vi "Open Connection to All - String Type Array.vi"(8 "Error In":errorcluster, 10 "Type array":string[](array[string]), 11 "URL array":string[](array[string])) -> (0 "Error Out":errorcluster, 2 "Error Status":bool, 3 "Array of SV Refnums":refnum<k21>[](array[refnum]))   [LabVIEW 2014]
doc: "<B>Copyright</B>: (c) 2015 MHWirth. All rights reserved.\n\nThis VI opens connection to all shared variables that are specified using URL and Type arrays.\n\nIf the type is unknown (Error 7001) or read variable function is errorenous, the loop stops and Error Status is True."
panel:
  out "Status":string
  out "Number of Deployed SV":i32
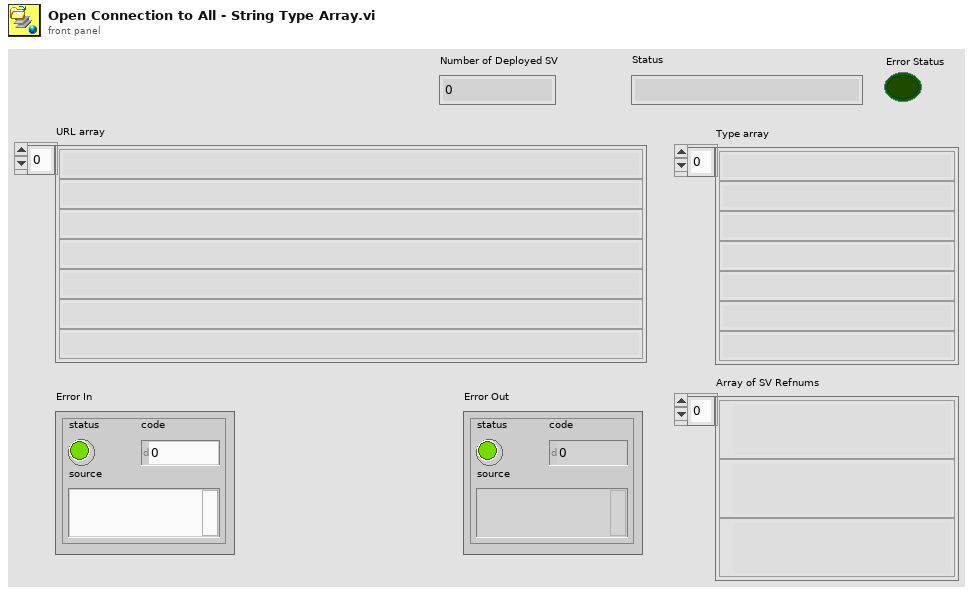
[diagram p1: front panel]
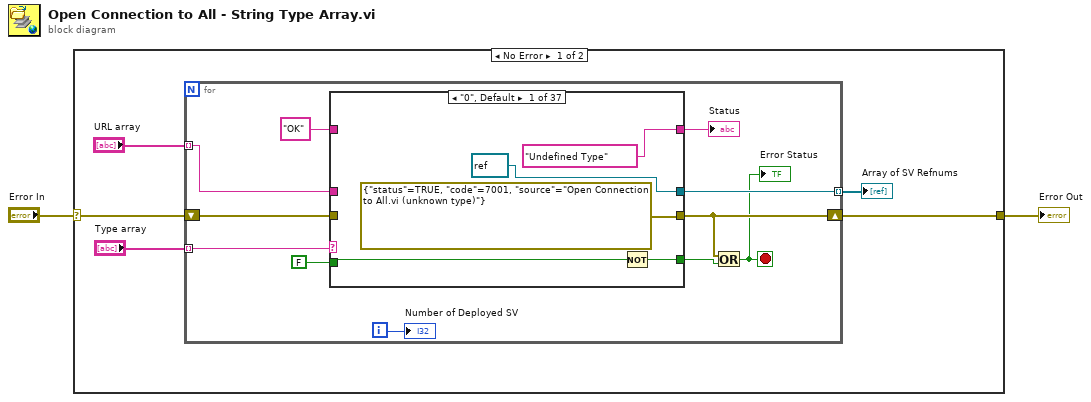
[diagram p0: block diagram]
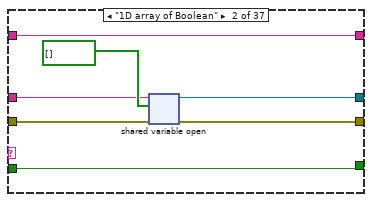
[diagram p2: hidden frame]
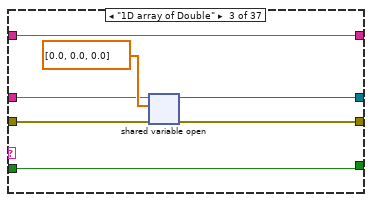
[diagram p3: hidden frame]
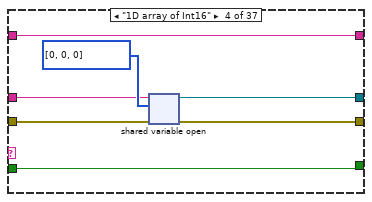
[diagram p4: hidden frame]
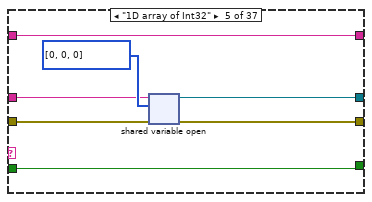
[diagram p5: hidden frame]
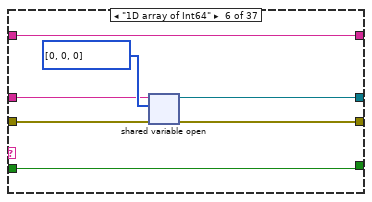
[diagram p6: hidden frame]
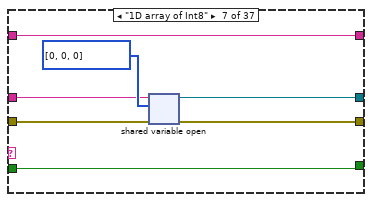
[diagram p7: hidden frame]
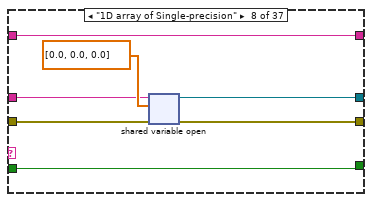
[diagram p8: hidden frame]
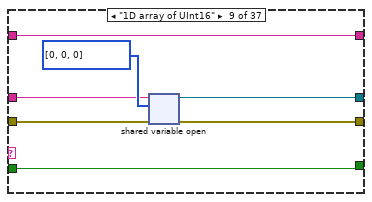
[diagram p9: hidden frame]
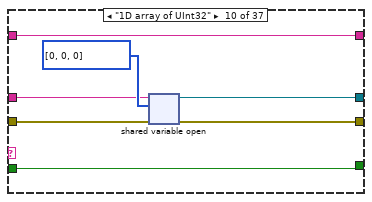
[diagram p10: hidden frame]
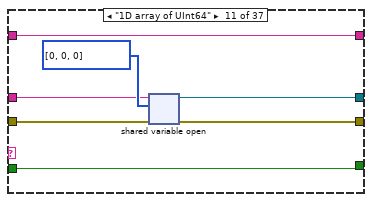
[diagram p11: hidden frame]
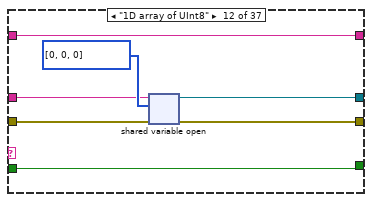
[diagram p12: hidden frame]
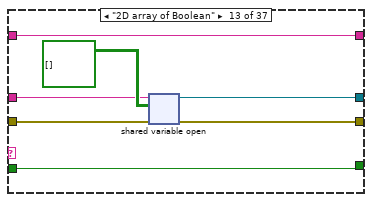
[diagram p13: hidden frame]
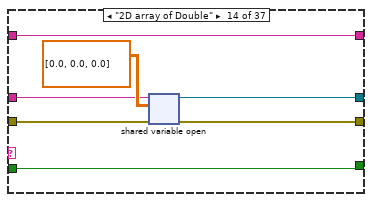
[diagram p14: hidden frame]
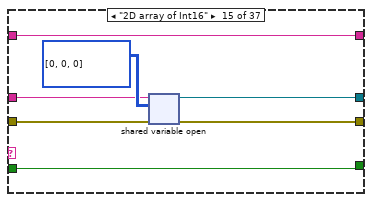
[diagram p15: hidden frame]
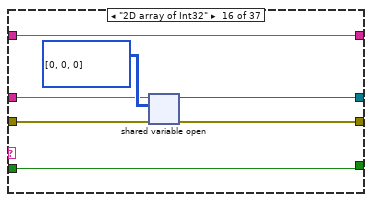
[diagram p16: hidden frame]
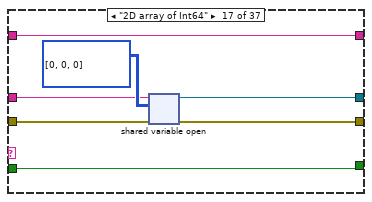
[diagram p17: hidden frame]
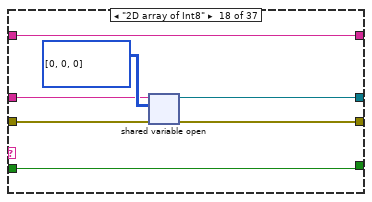
[diagram p18: hidden frame]
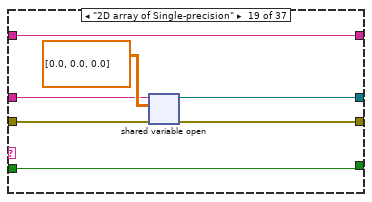
[diagram p19: hidden frame]
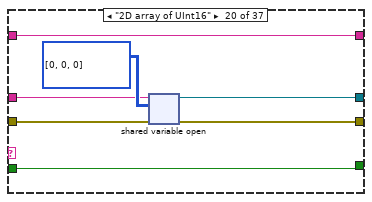
[diagram p20: hidden frame]
diagram:
  n1 = case shown="No Error" "Error In" {
    selector: "Error In" -> [w7 w276]
    tunnel: [w6 w276] -> w1
    frame No Error {
      n2 = for {
        shift-right: [w9] -> w6
        shift-left: w7 -> [w18]
        tunnel: "Type array" -> [w13] mode=indexing
        tunnel: "URL array" -> [w12] mode=indexing
        tunnel: [w11] -> w3 mode=indexing
        i -> [w17]
        stop <- w8 stop-if-true
        n3 = case shown="\"0\", Default" w13 {
          tunnel: w18 -> [_ w29 w36 w43 w50 w57 w64 w71 w78 w85 w92 w99 w106 w113 w120 w127 w134 w141 w148 w155 w162 w169 w176 w183 w191 w197 w204 w211 w218 w225 w232 w239 w246 w253 w260 w267 w274]
          tunnel: [errorcluster {"status"=TRUE, "code"=7001, "source"="Open Connection to All.vi (unknown type)"} ("error constant") w26 w32 w40 w47 w54 w61 w68 w75 w82 w89 w96 w103 w110 w117 w124 w131 w138 w145 w152 w159 w166 w173 w180 w187 w194 w201 w208 w215 w222 w229 w236 w243 w250 w257 w264 w271] -> w9
          tunnel: ["Undefined Type" w28 w35 w42 w49 w56 w63 w70 w77 w84 w91 w98 w105 w112 w119 w126 w133 w140 w147 w154 w161 w168 w175 w182 w190 w196 w203 w210 w217 w224 w231 w238 w245 w252 w259 w266 w273] -> w16
          tunnel: "OK" -> [_ w28 w35 w42 w49 w56 w63 w70 w77 w84 w91 w98 w105 w112 w119 w126 w133 w140 w147 w154 w161 w168 w175 w182 w190 w196 w203 w210 w217 w224 w231 w238 w245 w252 w259 w266 w273]
          tunnel: FALSE -> [w22 w27 w34 w41 w48 w55 w62 w69 w76 w83 w90 w97 w104 w111 w118 w125 w132 w139 w146 w153 w160 w167 w174 w181 w189 w195 w202 w209 w216 w223 w230 w237 w244 w251 w258 w265 w272]
          tunnel: [w21 w27 w34 w41 w48 w55 w62 w69 w76 w83 w90 w97 w104 w111 w118 w125 w132 w139 w146 w153 w160 w167 w174 w181 w189 w195 w202 w209 w216 w223 w230 w237 w244 w251 w258 w265 w272] -> w10
          tunnel: w12 -> [_ w25 w33 w39 w46 w53 w60 w67 w74 w81 w88 w95 w102 w109 w116 w123 w130 w137 w144 w151 w158 w165 w172 w179 w186 w193 w200 w207 w214 w221 w228 w235 w242 w249 w256 w263 w270]
          tunnel: [refnum<k21> refnum w24 w31 w38 w45 w52 w59 w66 w73 w80 w87 w94 w101 w108 w115 w122 w129 w136 w143 w150 w157 w164 w171 w178 w185 w192 w199 w206 w213 w220 w227 w234 w241 w248 w255 w262 w269] -> w11
          frame "0", Default {
            n4 = Not(x=w22) -> (.not. x?=w21:bool)
          }
          frame "1D array of Boolean" {
            n5 = shared-variable-open(w25, w29, bool[] []) -> (w24:refnum<k21>, w26:errorcluster)  [unwired: 1 in]
          }
          frame "1D array of Double" {
            n6 = shared-variable-open(w33, w36, dbl[] [0.0, 0.0, 0.0]) -> (w31:refnum<k21>, w32:errorcluster)  [unwired: 1 in]
          }
          frame "1D array of Int16" {
            n7 = shared-variable-open(w39, w43, i16[] [0, 0, 0]) -> (w38:refnum<k21>, w40:errorcluster)  [unwired: 1 in]
          }
          frame "1D array of Int32" {
            n8 = shared-variable-open(w46, w50, i32[] [0, 0, 0]) -> (w45:refnum<k21>, w47:errorcluster)  [unwired: 1 in]
          }
          frame "1D array of Int64" {
            n9 = shared-variable-open(w53, w57, i64[] [0, 0, 0]) -> (w52:refnum<k21>, w54:errorcluster)  [unwired: 1 in]
          }
          frame "1D array of Int8" {
            n10 = shared-variable-open(w60, w64, i8[] [0, 0, 0]) -> (w59:refnum<k21>, w61:errorcluster)  [unwired: 1 in]
          }
          frame "1D array of Single-precision" {
            n11 = shared-variable-open(w67, w71, sgl[] [0.0, 0.0, 0.0]) -> (w66:refnum<k21>, w68:errorcluster)  [unwired: 1 in]
          }
          frame "1D array of UInt16" {
            n12 = shared-variable-open(w74, w78, u16[] [0, 0, 0]) -> (w73:refnum<k21>, w75:errorcluster)  [unwired: 1 in]
          }
          frame "1D array of UInt32" {
            n13 = shared-variable-open(w81, w85, u32[] [0, 0, 0]) -> (w80:refnum<k21>, w82:errorcluster)  [unwired: 1 in]
          }
          frame "1D array of UInt64" {
            n14 = shared-variable-open(w88, w92, u64[] [0, 0, 0]) -> (w87:refnum<k21>, w89:errorcluster)  [unwired: 1 in]
          }
          frame "1D array of UInt8" {
            n15 = shared-variable-open(w95, w99, u8[] [0, 0, 0]) -> (w94:refnum<k21>, w96:errorcluster)  [unwired: 1 in]
          }
          frame "2D array of Boolean" {
            n16 = shared-variable-open(w102, w106, bool[][] []) -> (w101:refnum<k21>, w103:errorcluster)  [unwired: 1 in]
          }
          frame "2D array of Double" {
            n17 = shared-variable-open(w109, w113, dbl[][] [[0.0, 0.0, 0.0]]) -> (w108:refnum<k21>, w110:errorcluster)  [unwired: 1 in]
          }
          frame "2D array of Int16" {
            n18 = shared-variable-open(w116, w120, i16[][] [[0, 0, 0]]) -> (w115:refnum<k21>, w117:errorcluster)  [unwired: 1 in]
          }
          frame "2D array of Int32" {
            n19 = shared-variable-open(w123, w127, i32[][] [[0, 0, 0]]) -> (w122:refnum<k21>, w124:errorcluster)  [unwired: 1 in]
          }
          frame "2D array of Int64" {
            n20 = shared-variable-open(w130, w134, i64[][] [[0, 0, 0]]) -> (w129:refnum<k21>, w131:errorcluster)  [unwired: 1 in]
          }
          frame "2D array of Int8" {
            n21 = shared-variable-open(w137, w141, i8[][] [[0, 0, 0]]) -> (w136:refnum<k21>, w138:errorcluster)  [unwired: 1 in]
          }
          frame "2D array of Single-precision" {
            n22 = shared-variable-open(w144, w148, sgl[][] [[0.0, 0.0, 0.0]]) -> (w143:refnum<k21>, w145:errorcluster)  [unwired: 1 in]
          }
          frame "2D array of UInt16" {
            n23 = shared-variable-open(w151, w155, u16[][] [[0, 0, 0]]) -> (w150:refnum<k21>, w152:errorcluster)  [unwired: 1 in]
          }
          frame "2D array of UInt32" {
            n24 = shared-variable-open(w158, w162, u32[][] [[0, 0, 0]]) -> (w157:refnum<k21>, w159:errorcluster)  [unwired: 1 in]
          }
          frame "2D array of UInt64" {
            n25 = shared-variable-open(w165, w169, u64[][] [[0, 0, 0]]) -> (w164:refnum<k21>, w166:errorcluster)  [unwired: 1 in]
          }
          frame "2D array of UInt8" {
            n26 = shared-variable-open(w172, w176, u8[][] [[0, 0, 0]]) -> (w171:refnum<k21>, w173:errorcluster)  [unwired: 1 in]
          }
          frame "Boolean" {
            n27 = shared-variable-open(w179, w183, FALSE) -> (w178:refnum<k21>, w180:errorcluster)  [unwired: 1 in]
          }
          frame "String" {
            n28 = shared-variable-open(w186, w191, "dummy") -> (w185:refnum<k21>, w187:errorcluster)  [unwired: 1 in]
          }
          frame "Double" {
            n29 = shared-variable-open(w193, w197, 0.001) -> (w192:refnum<k21>, w194:errorcluster)  [unwired: 1 in]
          }
          frame "Fixed Point - signed" {
            n30 = shared-variable-open(w200, w204, fxp<+/-,32,16> 0.001007080078125) -> (w199:refnum<k21>, w201:errorcluster)  [unwired: 1 in]
          }
          frame "Fixed Point - unsigned" {
            n31 = shared-variable-open(w207, w211, fxp<+,32,16> 0.001007080078125) -> (w206:refnum<k21>, w208:errorcluster)  [unwired: 1 in]
          }
          frame "Int16" {
            n32 = shared-variable-open(w214, w218, i16 0) -> (w213:refnum<k21>, w215:errorcluster)  [unwired: 1 in]
          }
          frame "Int32" {
            n33 = shared-variable-open(w221, w225, 0) -> (w220:refnum<k21>, w222:errorcluster)  [unwired: 1 in]
          }
          frame "Int64" {
            n34 = shared-variable-open(w228, w232, i64 0) -> (w227:refnum<k21>, w229:errorcluster)  [unwired: 1 in]
          }
          frame "Int8" {
            n35 = shared-variable-open(w235, w239, i8 0) -> (w234:refnum<k21>, w236:errorcluster)  [unwired: 1 in]
          }
          frame "Single-precision" {
            n36 = shared-variable-open(w242, w246, sgl 0.001) -> (w241:refnum<k21>, w243:errorcluster)  [unwired: 1 in]
          }
          frame "UInt16" {
            n37 = shared-variable-open(w249, w253, u16 0) -> (w248:refnum<k21>, w250:errorcluster)  [unwired: 1 in]
          }
          frame "UInt32" {
            n38 = shared-variable-open(w256, w260, u32 0) -> (w255:refnum<k21>, w257:errorcluster)  [unwired: 1 in]
          }
          frame "UInt64" {
            n39 = shared-variable-open(w263, w267, u64 0) -> (w262:refnum<k21>, w264:errorcluster)  [unwired: 1 in]
          }
          frame "UInt8" {
            n40 = shared-variable-open(w270, w274, u8 0) -> (w269:refnum<k21>, w271:errorcluster)  [unwired: 1 in]
          }
        }
        "Status" <- w16
        n41 = Or(x=w9, y=w10) -> (x .or. y?=w8:bool)
        "Error Status" <- w8
        "Number of Deployed SV" <- w17
      }
      "Array of SV Refnums" <- w3
    }
    frame Error {
    }
  }
  "Error Out" <- w1
